vi "Enable or disable control or indicators.vi"(7 "Enable (T)/Disable&GrayOut (F)":bool, 8 "error in (no error)":errorcluster, 11 "aray of references in":refnum<vi>[](array[refnum])) -> (0 "error out":errorcluster, 3 "Array of references dup":refnum<vi>[](array[refnum]))   [LabVIEW 2020, in "ATM.lvlib"]
doc: "This VI is meant to enable o disable controls/indicators"
uses:
  ATM.lvlib
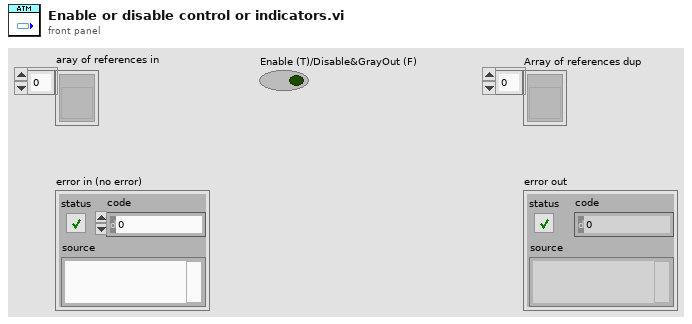
[diagram p1: front panel]
types:
  T1 = enum8{"Enabled", "Disabled", "Disabled and Grayed Out"}
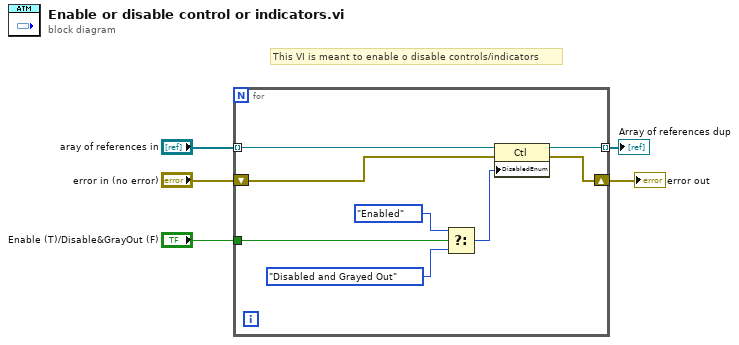
[diagram p0: block diagram]
diagram:
  # "This VI is meant to enable o disable controls/indicators"
  n1 = for {
    tunnel: "Enable (T)/Disable&GrayOut (F)" -> [w9]
    shift-right: [w12] -> w4
    shift-left: "error in (no error)" -> [w13]
    tunnel: "aray of references in" -> [w7] mode=indexing
    tunnel: [w6] -> w1 mode=indexing
    n2 = Select(t=T1."Enabled" ("Disabled"), s=w9, f=T1."Disabled and Grayed Out" ("Disabled")) -> (s? t:f=w8:T1)
    n3 = property class="Ctl"(reference=w7, error in=w13, "DisabledEnum"=w8) -> (reference out=w6:refnum<vi>, error out=w12:errorcluster)
  }
  "error out" <- w4
  "Array of references dup" <- w1
